vi "Set Config.vi"(8 "error in (no error)":errorcluster, 10 "Config":T1={"Execution View Required?"=TRUE, "Sequence File View Required?"=FALSE}, 11 "teststand-api in":refnum<class "teststand-api.lvclass">) -> (0 "error out":errorcluster, 3 "teststand-api out":refnum<class "teststand-api.lvclass">)   [LabVIEW 2014, in "teststand-api.lvlib" / "teststand-api.lvclass"]
uses:
  teststand-api.lvclass
  Config Argument--cluster.ctl
  teststand-api.lvclass/teststand-api.ctl
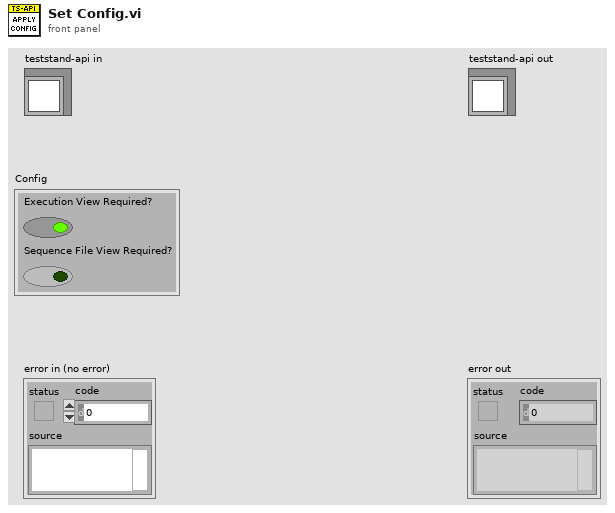
[diagram p1: front panel]
types:
  T1 = typedef "teststand-api.lvlib/teststand-api.lvclass/Config Argument--cluster.ctl" = cluster{"Execution View Required?":bool, "Sequence File View Required?":bool}
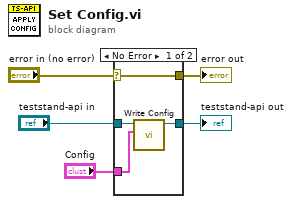
[diagram p0: block diagram]
diagram:
  n1 = case shown="No Error" "error in (no error)" {
    selector: "error in (no error)" -> [w9 w11]
    tunnel: [w9 w11] -> w4
    tunnel: [w7 w10] -> w2
    tunnel: "teststand-api in" -> [w8 w10]
    tunnel: "Config" -> [w6 _]
    frame No Error {
      n2 = call "Write Config.vi"("Config"=w6, "teststand-api in"=w8) -> ("teststand-api out"=w7:refnum<class "teststand-api.lvclass">)  [unwired: 8 in, 1 out]
    }
    frame Error {
    }
  }
  "error out" <- w4
  "teststand-api out" <- w2
